vi "scales uv-vis.vi"() -> ()   [LabVIEW 2010]
panel:
  out "Array 2":ext[](array[numeric])
  out "Array":ext[](array[numeric])
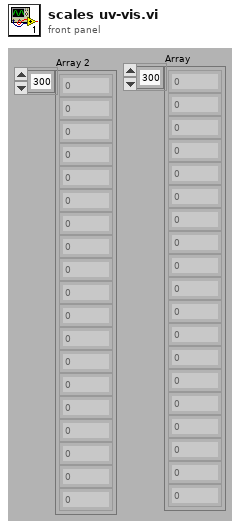
[diagram p1: front panel]
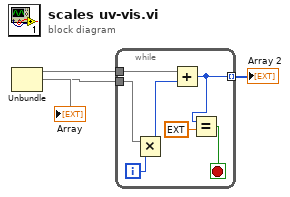
[diagram p0: block diagram]
diagram:
  n1 = Unbundle() -> (w5:cluster{ext, ext, ext[]}, w3, w2, →"Array")
  n2 = while {
    tunnel: w3 -> [w12]
    tunnel: w2 -> [w10]
    tunnel: [w7] -> w1 mode=indexing
    i -> [w11]
    stop <- w8 stop-if-true
    n3 = Multiply(x=w10, y=w11) -> (x*y=w9:i32)
    n4 = Add(x=w12, y=w9) -> (x+y=w7:i32)
    n5 = Equal?(x=w7, y=ext 820.0) -> (x = y?=w8:bool)
  }
  "Array 2" <- w1
